vi "example_09_combo_box_input.vi"() -> ()   [LabVIEW 2015, in "lv-dialog.lvlib" / "v1.lvlib"]
uses:
  v1.lvlib
  public/_controls/selection.ctl
  public/class/v1.lvclass
panel:
  in  "custom_entry":bool
  in  "combo_box []":string[](array[string])=["Option 1", "Option 2", "Option 3"]
  in  "boolean_text_2":string="Cancel"
  in  "boolean_text_1":string="Select"
  in  "dialog_text":string="Choose an option"
  out "value":string
  out "error out":errorcluster
  out "dialog_selection":T1
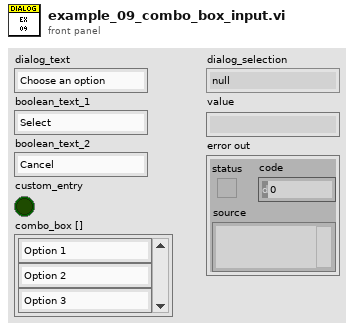
[diagram p1: front panel]
types:
  T1 = typedef "lv-dialog.lvlib/v1.lvlib/selection.ctl" = enum16{"null", "panel_closed", "button_1", "button_2", "button_3", "cancelled"}
  T2 = cluster{"dialog_text":string, "boolean_text_1":string, "boolean_text_2":string, "combo_box []":string[], "custom_entry":bool}
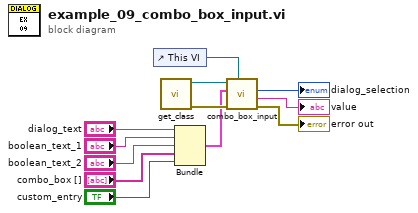
[diagram p0: block diagram]
diagram:
  n1 = control-ref of="This VI"() -> (w12:refnum<vi>)
  n2 = call "get_class.vi"() -> ("error out"=w8:errorcluster, "class"=w9:refnum<class "v1.lvclass">)  [unwired: 10 in]
  n3 = Bundle("dialog_text"="dialog_text", "boolean_text_1"="boolean_text_1", "boolean_text_2"="boolean_text_2", "combo_box []"="combo_box []", "custom_entry"="custom_entry") -> (w2:T2)  [unwired: 1 in]
  n4 = call-dynamic "combo_box_input.vi"("callee"=w12, "error in (no error)"=w8, "configuration"=w2, "v1 in"=w9) -> ("error out"=→"error out":errorcluster, "value"=→"value":string, "dialog_selection"=→"dialog_selection":T1)  [unwired: 4 in, 1 out]
